vi "显示 (子VI).vi"(10 "数值":dbl) -> (3 "簇 个位":T1)   [LabVIEW 2020]
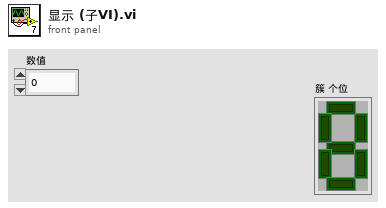
[diagram p1: front panel]
types:
  T1 = cluster{"布尔":bool, "布尔 2":bool, "布尔 3":bool, "布尔 4":bool, "布尔 5":bool, "布尔 6":bool, "布尔 7":bool}
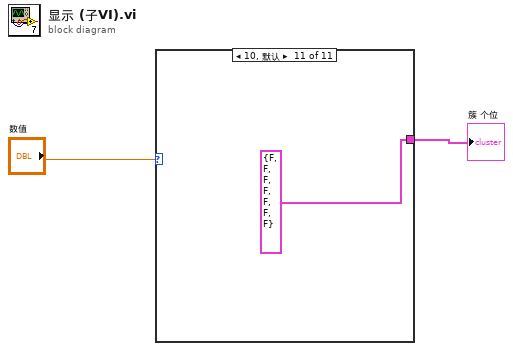
[diagram p0: block diagram]
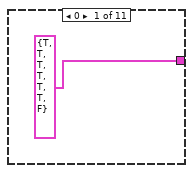
[diagram p2: hidden frame]
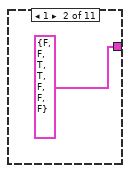
[diagram p3: hidden frame]
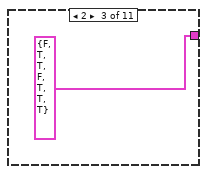
[diagram p4: hidden frame]
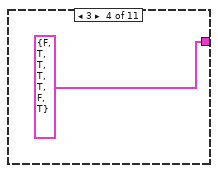
[diagram p5: hidden frame]
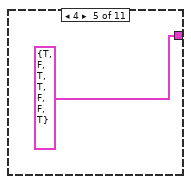
[diagram p6: hidden frame]
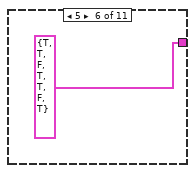
[diagram p7: hidden frame]
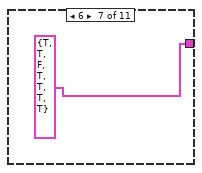
[diagram p8: hidden frame]
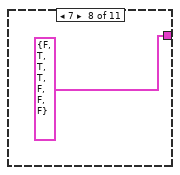
[diagram p9: hidden frame]
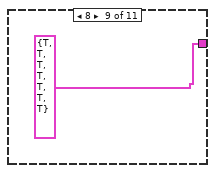
[diagram p10: hidden frame]
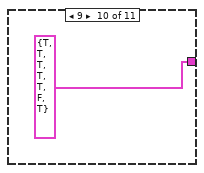
[diagram p11: hidden frame]
diagram:
  n1 = case shown="10, 默认" "数值" {
    tunnel: [T1 {"布尔"=TRUE, "布尔 2"=TRUE, "布尔 3"=TRUE, "布尔 4"=TRUE, "布尔 5"=TRUE, "布尔 6"=TRUE, "布尔 7"=FALSE} T1 {"布尔"=FALSE, "布尔 2"=FALSE, "布尔 3"=TRUE, "布尔 4"=TRUE, "布尔 5"=FALSE, "布尔 6"=FALSE, "布尔 7"=FALSE} T1 {"布尔"=FALSE, "布尔 2"=TRUE, "布尔 3"=TRUE, "布尔 4"=FALSE, "布尔 5"=TRUE, "布尔 6"=TRUE, "布尔 7"=TRUE} T1 {"布尔"=FALSE, "布尔 2"=TRUE, "布尔 3"=TRUE, "布尔 4"=TRUE, "布尔 5"=TRUE, "布尔 6"=FALSE, "布尔 7"=TRUE} T1 {"布尔"=TRUE, "布尔 2"=FALSE, "布尔 3"=TRUE, "布尔 4"=TRUE, "布尔 5"=FALSE, "布尔 6"=FALSE, "布尔 7"=TRUE} T1 {"布尔"=TRUE, "布尔 2"=TRUE, "布尔 3"=FALSE, "布尔 4"=TRUE, "布尔 5"=TRUE, "布尔 6"=FALSE, "布尔 7"=TRUE} T1 {"布尔"=TRUE, "布尔 2"=TRUE, "布尔 3"=FALSE, "布尔 4"=TRUE, "布尔 5"=TRUE, "布尔 6"=TRUE, "布尔 7"=TRUE} T1 {"布尔"=FALSE, "布尔 2"=TRUE, "布尔 3"=TRUE, "布尔 4"=TRUE, "布尔 5"=FALSE, "布尔 6"=FALSE, "布尔 7"=FALSE} T1 {"布尔"=TRUE, "布尔 2"=TRUE, "布尔 3"=TRUE, "布尔 4"=TRUE, "布尔 5"=TRUE, "布尔 6"=TRUE, "布尔 7"=TRUE} T1 {"布尔"=TRUE, "布尔 2"=TRUE, "布尔 3"=TRUE, "布尔 4"=TRUE, "布尔 5"=TRUE, "布尔 6"=FALSE, "布尔 7"=TRUE} T1 {"布尔"=FALSE, "布尔 2"=FALSE, "布尔 3"=FALSE, "布尔 4"=FALSE, "布尔 5"=FALSE, "布尔 6"=FALSE, "布尔 7"=FALSE}] -> w1
    frame 0 {
    }
    frame 1 {
    }
    frame 2 {
    }
    frame 3 {
    }
    frame 4 {
    }
    frame 5 {
    }
    frame 6 {
    }
    frame 7 {
    }
    frame 8 {
    }
    frame 9 {
    }
    frame 10, Default {
    }
  }
  "簇 个位" <- w1
